vi "Main_Run.vi"(8 "error in (no error)":errorcluster, 9 "Spray type":u16, 10 "Step type":u16, 11 "VISA resource name":refnum<visa-resource-name>) -> (0 "error out":errorcluster, 3 "VISA resource name out":refnum<visa-resource-name>)   [LabVIEW 2015]
panel:
  in  "milliseconds spraying":u32
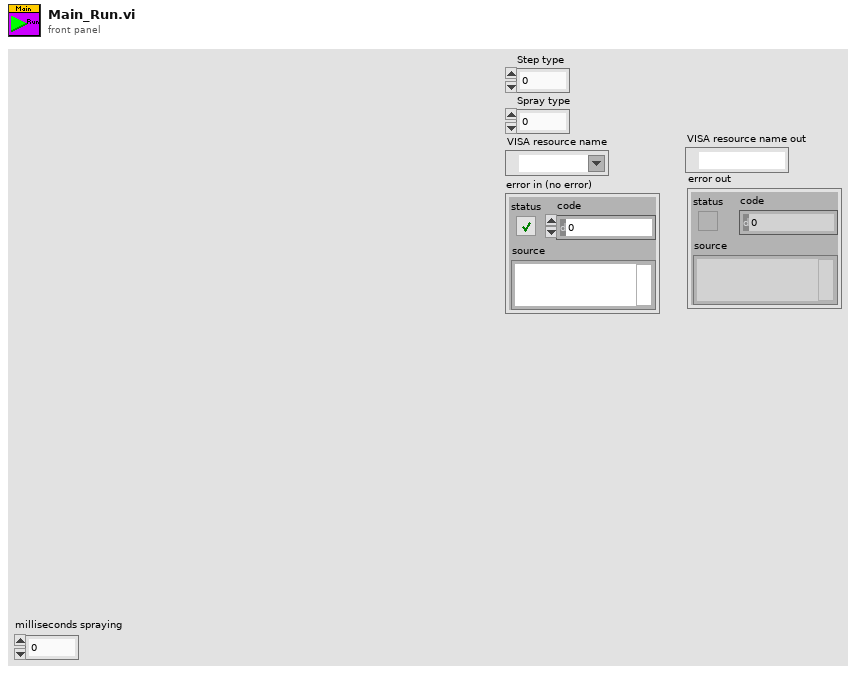
[diagram p1: front panel]
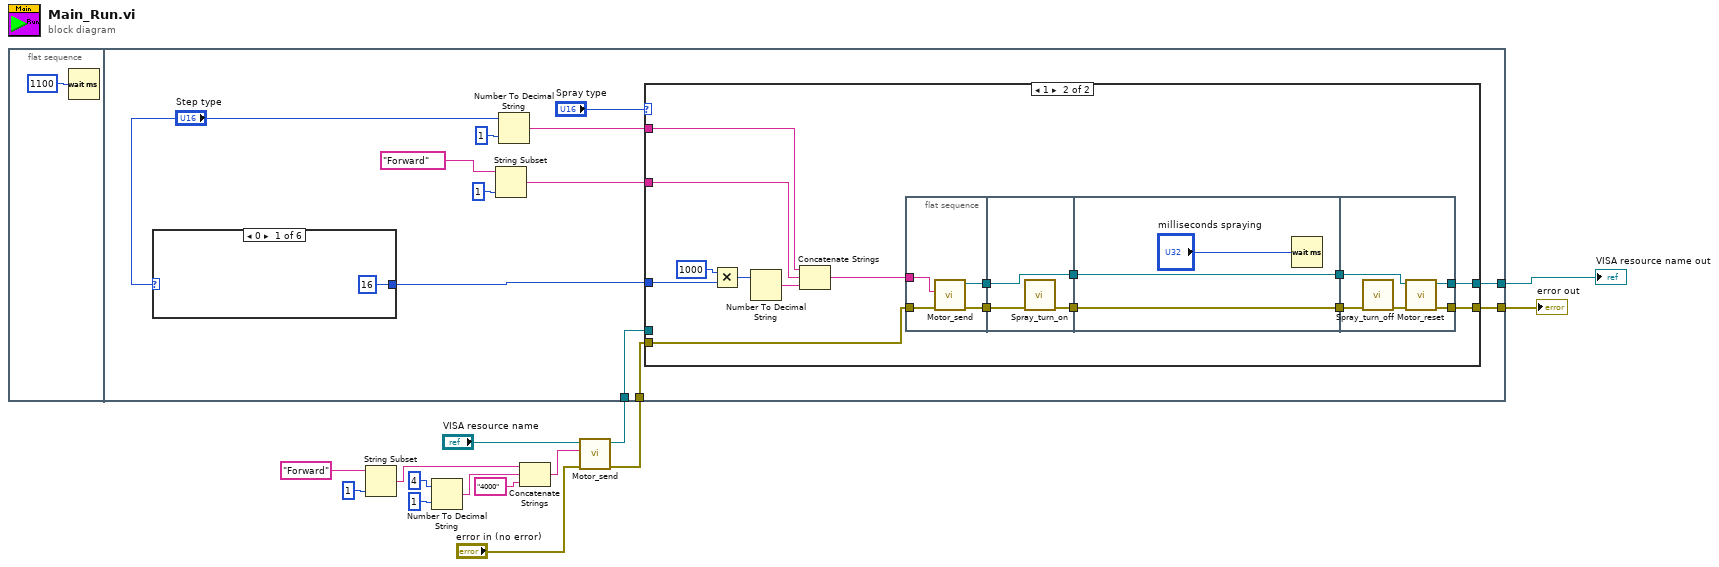
[diagram p0: block diagram]
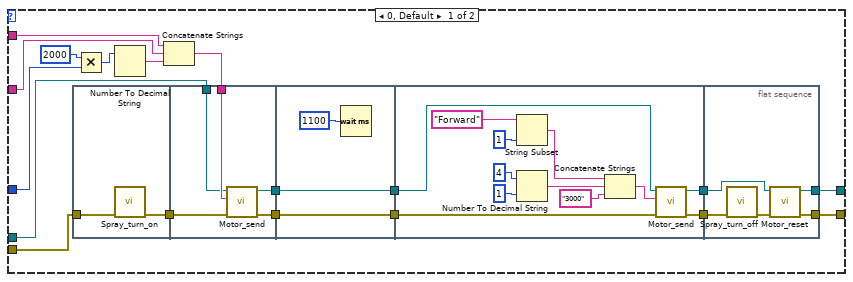
[diagram p2: hidden frame]
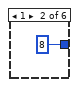
[diagram p3: hidden frame]
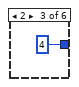
[diagram p4: hidden frame]
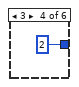
[diagram p5: hidden frame]
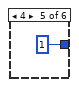
[diagram p6: hidden frame]
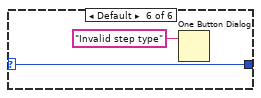
[diagram p7: hidden frame]
diagram:
  n1 = flat-sequence {
    tunnel: w5 -> [w21]
    tunnel: w6 -> [w18]
    tunnel: [w17] -> w2
    tunnel: [w16] -> w1
    frame #0 {
      n2 = Wait (ms)(milliseconds to wait=u32 1100) -> ()  [unwired: 1 out]
    }
    frame #1 {
      n3 = case shown="0" "Step type" {
        selector: "Step type" -> [_ _ _ _ _ w109]
        tunnel: [16 8 4 2 1 w109] -> w24
        frame 0 {
        }
        frame 1 {
        }
        frame 2 {
        }
        frame 3 {
        }
        frame 4 {
        }
        frame Default {
          n4 = One Button Dialog(message="Invalid step type") -> ()  [unwired: 1 in, 1 out]
        }
      }
      n5 = String Subset(string="Forward" ("Direction"), length (rest)=1) -> (substring=w22:string)  [unwired: 1 in]
      n6 = Number To Decimal String(number="Step type", width (-)=1) -> (decimal integer string=w23:string)
      n7 = case shown="1" "Spray type" {
        tunnel: w24 -> [w44 w83]
        tunnel: w23 -> [w43 w85]
        tunnel: w22 -> [w42 w84]
        tunnel: w21 -> [w40 w82]
        tunnel: w18 -> [w31 _]
        tunnel: [w28 w73] -> w17
        tunnel: [w30 w77] -> w16
        frame 0, Default {
          n8 = flat-sequence {
            tunnel: w40 -> [w47]
            tunnel: [w46] -> w33
            tunnel: [w52] -> w37
            tunnel: [w51] -> w35
            tunnel: w34 -> [w50]
            tunnel: w33 -> [w49]
            tunnel: w31 -> [w48]
            tunnel: [w54] -> w38
            tunnel: w37 -> [w54]
            tunnel: [w53] -> w36
            tunnel: w35 -> [w53]
            tunnel: w38 -> [w60]
            tunnel: w36 -> [w59]
            tunnel: [w57] -> w32
            tunnel: [w56] -> w29
            tunnel: w32 -> [w72]
            tunnel: [w70] -> w30
            tunnel: w29 -> [w69]
            tunnel: [w68] -> w28
            frame #0 {
              n9 = call "Spray_turn_on.vi"("error in (no error)"=w47) -> ("error out"=w46:errorcluster)  [unwired: 10 in]
            }
            frame #1 {
              n10 = call "Motor_send.vi"("error in (no error)"=w49, "String"=w50, "VISA resource name"=w48) -> ("error out"=w51:errorcluster, "VISA resource name out"=w52:refnum<visa-resource-name>)  [unwired: 7 in]
            }
            frame #2 {
              n11 = Wait (ms)(milliseconds to wait=u32 1100) -> ()  [unwired: 1 out]
            }
            frame #3 {
              n12 = String Subset(string="Forward", length (rest)=1) -> (substring=w61:string)  [unwired: 1 in]
              n13 = Number To Decimal String(number=4, width (-)=1) -> (decimal integer string=w65:string)
              n14 = Concatenate Strings(w61, w65, "3000") -> (w58:string)
              n15 = call "Motor_send.vi"("error in (no error)"=w59, "String"=w58, "VISA resource name"=w60) -> ("error out"=w57:errorcluster, "VISA resource name out"=w56:refnum<visa-resource-name>)  [unwired: 7 in]
            }
            frame #4 {
              n16 = call "Spray_turn_off.vi"("error in (no error)"=w72) -> ("error out"=w71:errorcluster)  [unwired: 10 in]
              n17 = call "Motor_reset.vi"("error in (no error)"=w71, "VISA resource name"=w69) -> ("error out"=w70:errorcluster, "VISA resource name out"=w68:refnum<visa-resource-name>)  [unwired: 8 in]
            }
          }
          n18 = Multiply(x=2000, y=w44) -> (x*y=w41:i32)
          n19 = Number To Decimal String(number=w41) -> (decimal integer string=w39:string)  [unwired: 1 in]
          n20 = Concatenate Strings(w43, w42, w39) -> (w34:string)
        }
        frame 1 {
          n21 = Multiply(x=1000, y=w83) -> (x*y=w87:i32)
          n22 = Number To Decimal String(number=w87) -> (decimal integer string=w86:string)  [unwired: 1 in]
          n23 = Concatenate Strings(w85, w84, w86) -> (w81:string)
          n24 = flat-sequence {
            tunnel: w82 -> [w92]
            tunnel: w81 -> [w91]
            tunnel: [w90] -> w80
            tunnel: [w89] -> w74
            tunnel: w80 -> [w95]
            tunnel: [w94] -> w79
            tunnel: [w93] -> w75
            tunnel: w74 -> [w93]
            tunnel: w79 -> [w97]
            tunnel: [w97] -> w78
            tunnel: [w96] -> w76
            tunnel: w75 -> [w96]
            tunnel: w78 -> [w103]
            tunnel: [w102] -> w77
            tunnel: w76 -> [w100]
            tunnel: [w99] -> w73
            frame #0 {
              n25 = call "Motor_send.vi"("error in (no error)"=w92, "String"=w91) -> ("error out"=w90:errorcluster, "VISA resource name out"=w89:refnum<visa-resource-name>)  [unwired: 8 in]
            }
            frame #1 {
              n26 = call "Spray_turn_on.vi"("error in (no error)"=w95) -> ("error out"=w94:errorcluster)  [unwired: 10 in]
            }
            frame #2 {
              n27 = Wait (ms)(milliseconds to wait="milliseconds spraying") -> ()  [unwired: 1 out]
            }
            frame #3 {
              n28 = call "Spray_turn_off.vi"("error in (no error)"=w103) -> ("error out"=w101:errorcluster)  [unwired: 10 in]
              n29 = call "Motor_reset.vi"("error in (no error)"=w101, "VISA resource name"=w100) -> ("error out"=w102:errorcluster, "VISA resource name out"=w99:refnum<visa-resource-name>)  [unwired: 8 in]
            }
          }
        }
      }
    }
  }
  n30 = String Subset(string="Forward", length (rest)=1) -> (substring=w11:string)  [unwired: 1 in]
  n31 = Number To Decimal String(number=4, width (-)=1) -> (decimal integer string=w12:string)
  n32 = Concatenate Strings(w11, w12, "4000") -> (w10:string)
  n33 = call "Motor_send.vi"("error in (no error)"="error in (no error)", "String"=w10, "VISA resource name"="VISA resource name") -> ("error out"=w5:errorcluster, "VISA resource name out"=w6:refnum<visa-resource-name>)  [unwired: 7 in]
  "VISA resource name out" <- w2
  "error out" <- w1
